vi "BuildModel.vi"(2 "Model Name":string="My_Model", 4 "3D Picture":refnum<vi>, 5 "urdf in":string) -> (0 "3D Picture":refnum<vi>(3d-picture), 1 "urdf out":string)   [LabVIEW 2010]
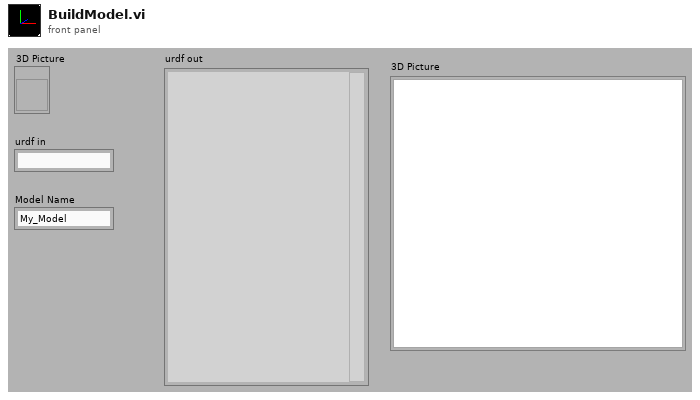
[diagram p1: front panel]
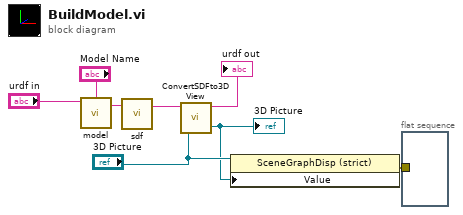
[diagram p0: block diagram]
diagram:
  n1 = call "model.vi"("Joints.urdf"="urdf in", "Name"="Model Name") -> ("urdf out"=w5:string)  [unwired: 2 in]
  n2 = call "sdf.vi"("assets"=w5) -> ("sdf out"=w6:string)  [unwired: 2 in]
  "urdf out" <- w6
  n3 = call "ConvertSDFto3DView.vi"("SceneGraphDisp Refnum"="3D Picture", "urdf"=w6) -> ("3D Picture"=w2:refnum<vi>)  [unwired: 1 out]
  "3D Picture" <- w2
  n4 = property class="SceneGraphDisp (strict)"(reference="3D Picture", "Value"=w2) -> (error out=w1:errorcluster)  [unwired: 1 in, 1 out]
  n5 = flat-sequence {
    tunnel: w1 -> [_]
    frame #0 {
    }
  }
